vi "testVideo.vi"() -> ()   [LabVIEW 2009, in "run.lvlib"]
uses:
  run.lvlib
panel:
  out "Image":T1(plugin-control)
  in  "stop":bool
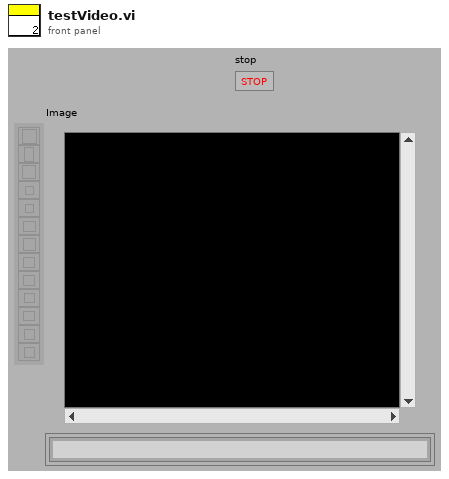
[diagram p1: front panel]
types:
  T1 = typedef "IMAQ Image.ctl" = refnum<image>
  T2 = typedef "Image Type" = u32
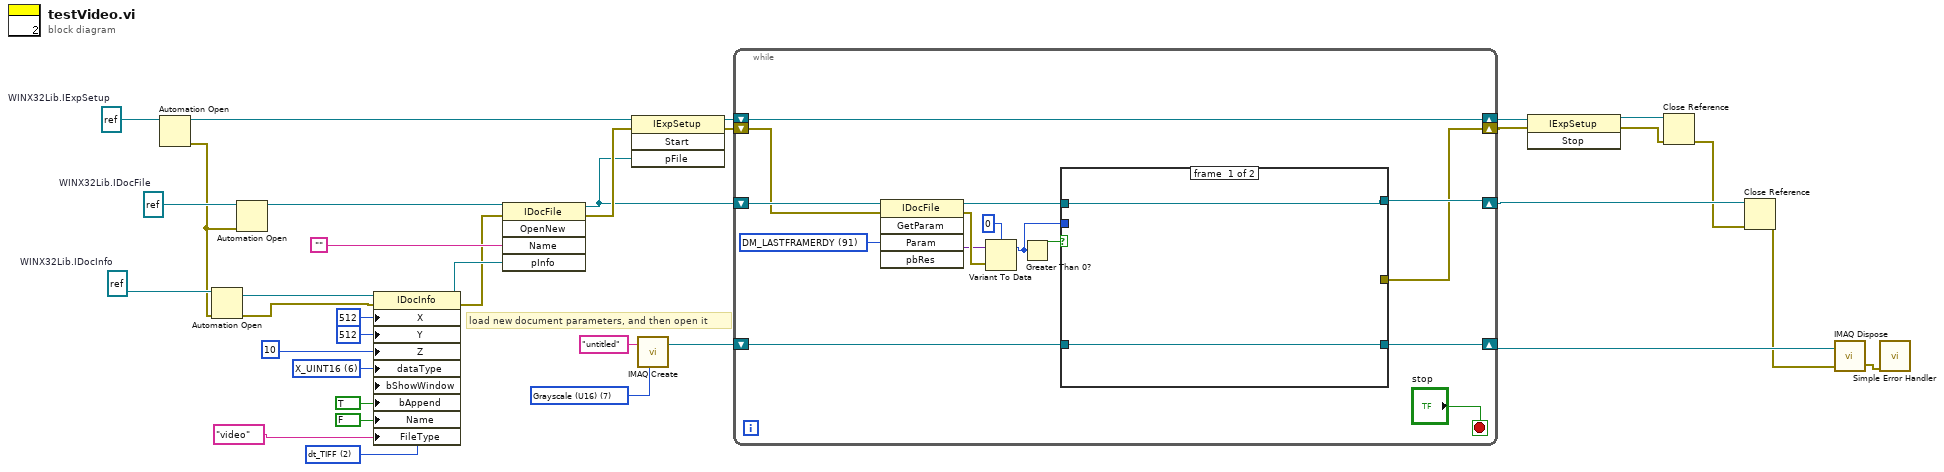
[diagram p0: block diagram]
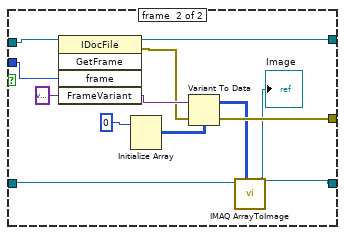
[diagram p2: hidden frame]
diagram:
  w10 = T2 7 items=["Grayscale (U8)", "Grayscale (I16)", "Grayscale (SGL)", "Complex (CSG)", "RGB (U32)", "HSL (U32)", "RGB (U64)", "Grayscale (U16)"] ("Image Type")
  w24 = refnum<k7> refnum  # WINX32Lib.IDocFile
  w28 = refnum<k7> refnum  # WINX32Lib.IDocInfo
  w31 = 6 items=["X_UNKNOWN"=0, "X_SHORT"=1, "X_LONG"=2, "X_FLOAT"=3, "X_DOUBLE"=4, "X_BYTE"=5, "X_UINT16"=6, "X_ULONG"=7, "X_LASTTYPE"=8, "X_ENUM"=9, "X_NODATATYPE"=10, "X_BOOL"=11, "X_CHAR_PTR"=13] ("dataType")
  w34 = 2 items=["dt_NONE", "dt_SPE", "dt_TIFF", "dt_TIF8", "dt_ASCII", "dt_NUMTYPES"] ("FileType")
  w35 = refnum<k7> refnum  # WINX32Lib.IExpSetup
  # "load new document parameters, and then open it"
  n1 = Automation Open(Automation Refnum=w35) -> (Automation Refnum=w17:refnum<k7>, error out=w23:errorcluster)  [unwired: 3 in]
  n2 = Automation Open(error in (no error)=w23, Automation Refnum=w28) -> (Automation Refnum=w27:refnum<k7>, error out=w26:errorcluster)  [unwired: 2 in]
  n3 = Automation Open(error in (no error)=w23, Automation Refnum=w24) -> (Automation Refnum=w21:refnum<k7>)  [unwired: 2 in, 1 out]
  n4 = property class="IDocInfo"(reference=w27, error in=w26, "X"=512, "Y"=512, "Z"=10, "dataType"=w31, "bShowWindow"=TRUE, "bAppend"=FALSE, "Name"="video", "FileType"=w34) -> (reference out=w20:refnum<k7>, error out=w19:errorcluster)
  n5 = invoke class="IDocFile" method="OpenNew"(reference=w21, error in=w19, "Name"="", "pInfo"=w20) -> (reference out=w13:refnum<k7>, error out=w14:errorcluster)  [unwired: 1 in, 3 out]
  n6 = invoke class="IExpSetup" method="Start"(reference=w17, error in=w14, "pFile"=w13) -> (reference out=w16:refnum<k7>, error out=w15:errorcluster)  [unwired: 1 in, 2 out]
  n7 = call "IMAQ Create"("Image Name"="untitled", "Image Type"=w10) -> ("New Image"=w11:T1)  [unwired: 3 in, 1 out]
  n8 = while {
    shift-right: [w39] -> w9
    shift-left: w16 -> [w39]
    shift-right: [w40] -> w8
    shift-left: w15 -> [w48]
    shift-right: [w41] -> w5
    shift-left: w13 -> [w50]
    shift-right: [w36] -> w3
    shift-left: w11 -> [w37]
    stop <- "stop" stop-if-true
    w49 = 91 items=["DM_XDIMDET"=1, "DM_YDIMDET"=2, "DM_TIMINGMODE"=3, "DM_EXPOSEC"=4, "DM_DETTYPE"=5, "DM_XDIM"=6, "DM_YDIM"=7, "DM_ASYNEN"=8, "DM_DATATYPE"=9, "DM_PIXELSIZE"=10, "DM_MINBLK"=11, "DM_NUMMINBLK"=12, "DM_ADCRATE"=13, "DM_ADCTYPE"=14, "DM_ADCRESOLUTION"=15, "DM_ADCBITADJUST"=16, "DM_GAIN"=17, "DM_GEOMETRIC"=18, "DM_CLEANS"=19, "DM_NUMSKPPERCLN"=20, "DM_FILEVERSION"=21, "DM_SWVERSION"=22, "DM_CONTROLLERTYPE"=23, "DM_NUMFRAMES"=24, "DM_MAXINTENSITY"=25, "DM_MININTENSITY"=26, "DM_SHUTTERTYPE"=27, "DM_SHUTTERCOMP"=28, "DM_READOUTMODE"=29, "DM_WINDOWSIZE"=30, "DM_CLKSPD"=31, "DM_KINTRIGMODE"=32, "DM_CLKSPD_us"=33, "DM_INTERFACETYPE"=34, "DM_NOT_IN_USE_0"=35, "DM_NOT_IN_USE_1"=36, "DM_NOT_IN_USE_2"=37, "DM_NOT_IN_USE_3"=38, "DM_NOT_IN_USE_4"=39, "DM_NOT_IN_USE_5"=40, "DM_COSMICAPPLIED"=41, "DM_COSMICTYPE"=42, "DM_COSMICTHRESHOLD"=43, "DM_BLEMISHAPPLIED"=44, "DM_FLATFIELDAPPLIED"=45, "DM_BACKGROUNDAPPLIED"=46, "DM_ACCUMS"=47, "DM_HWACCUMS"=48, "DM_NOT_IN_USE_6"=49, "DM_NOT_IN_USE_7"=50, "DM_NOT_IN_USE_8"=51, "DM_STORESYNC"=52, "DM_SWMADE"=53, "DM_FLATFIELDNAME"=54, "DM_BACKSUBNAME"=55, "DM_XLABEL"=56, "DM_YLABEL"=57, "DM_DLABEL"=58, "DM_FILEDATE"=59, "DM_BLEMISHFILE"=60, "DM_USERINFO"=61, "DM_USERCOMMENT1"=62, "DM_USERCOMMENT2"=63, "DM_USERCOMMENT3"=64, "DM_USERCOMMENT4"=65, "DM_USERCOMMENT5"=66, "DM_xCAL_OFFSET"=67, "DM_xCAL_FACTOR"=68, "DM_xCAL_CURR_UNIT"=69, "DM_xCAL_STRING"=70, "DM_xCAL_VALID"=71, "DM_xCAL_INPUT_UNIT"=72, "DM_xCAL_POLYNOM_UNIT"=73, "DM_xCAL_CALIB_COUNT"=74, "DM_xCAL_PXL_POS"=75, "DM_xCAL_PXL_VAL"=76, "DM_xCAL_POLYNOM_ORDER"=77, "DM_xCAL_COEFFS"=78, "DM_xCAL_LASERLINE"=79, "DM_xCAL_FILE_LABEL"=80, "DM_NUMROI"=81, "DM_ROI_STARTX"=82, "DM_ROI_ENDX"=83, "DM_ROI_GP_X"=84, "DM_ROI_STARTY"=85, "DM_ROI_ENDY"=86, "DM_ROI_GP_Y"=87, "DM_CONTROLLERNUM"=88, "DM_DEFAULTTYPE"=89, "DM_FRAMECOUNT"=90, "DM_LASTFRAMERDY"=91, "DM_FRAMEINPROS"=92, "DM_SCANCOUNT"=93, "DM_TEMPFLAG"=94, "DM_STOREFLAG"=95, "DM_FRAMESIZE"=96, "DM_ISDISPLAYED"=97, "DM_INUSE"=98, "DM_LASTVALUE"=99, "DM_STOREFLAGSAVE"=100, "DM_YTFLAG"=101, "DM_YT_AREAS_EQUS"=102, "DM_YT_POINTS_TAKEN"=103, "DM_FILENAME"=104, "DM_FILETITLE"=105, "DM_DOCTYPE"=106, "DM_NUMEXPREPEATS"=107, "DM_NUMEXPACCUMS"=108, "DM_UPDATEVIEWS"=109, "DM_PULSEFILENAME"=110, "DM_PULSEREPWIDTH"=111, "DM_PULSEREPDELAY"=112, "DM_CONTROLLERVERSION"=113, "DM_LOGICOUTPUT"=114, "DM_VIRTUALCHIPFLAG"=115, "DM_PULSERTYPE"=116, "DM_AMPHICAPLOWNOISE"=117, "DM_VCHIPXDIM"=118, "DM_VCHIPYDIM"=119, "DM_PIMAXUSED"=120, "DM_PIMAXMODE"=121, "DM_SHUTTERCONTROL"=122, "DM_ABSORBLIVE"=123, "DM_ABSORBMODE"=124, "DM_ABSORBSTRIPNUM"=125, "DM_THRESHOLDMINLIVE"=126, "DM_THRESHOLDMAXLIVE"=127, "DM_SPECAUTOSPECTROMODE"=128, "DM_SPECGLUEFLAG"=129, "DM_PULSERMODE"=130, "DM_PULSERONCHIPACCUMS"=131, "DM_PULSERREPEATEXP"=132, "DM_PULSESEQINCMODE"=133, "DM_ADCOFFSET"=134, "DM_ABSORBFILENAME"=135, "DM_NUMROISINEXPERIMENT"=136, "DM_SPECMIRRORLOCATION"=137, "DM_SPECSLITLOCATION"=138, "DM_SPECMIRRORPOS"=139, "DM_READOUTTIME"=140, "DM_DETTEMPERATURE"=141, "DM_DELAYTIME"=142, "DM_THRESHOLDMINVAL"=143, "DM_THRESHOLDMAXVAL"=144, "DM_SPECCENTERWLNM"=145, "DM_SPECGLUESTARTWLNM"=146, "DM_SPECGLUEENDWLNM"=147, "DM_SPECGLUEMINOVRLPNM"=148, "DM_SPECGLUEFINALRESNM"=149, "DM_PULSESEQSTARTWIDTH"=150, "DM_PULSESEQENDWIDTH"=151, "DM_PULSESEQSTARTDELAY"=152, "DM_PULSESEQENDDELAY"=153, "DM_SPECSLITPOS"=154, "DM_AUTOCLEANSACTIVE"=155, "DM_USECONTCLEANSINST"=156, "DM_CUSTOMCHIPFLAG"=157, "DM_XPREPIXELS"=158, "DM_XPOSTPIXELS"=159, "DM_YPREPIXELS"=160, "DM_YPOSTPIXELS"=161, "DM_CUSTOMTIMINGFLAG"=162, "DM_CANDOVIRTUALCHIPFLAG"=163, "DM_PIMAXGAIN"=164, "DM_PIMAX2NSBRDUSED"=165, "DM_TRIGGEREDMODEFLAG"=166, "DM_CONTINUOUSCLEANSFLAG"=167, "DM_EXTERNALTRIGGERFLAG"=168, "DM_EXPERIMENTTIMELOCAL"=169, "DM_EXPERIMENTTIMEUTC"=170, "DM_EXPOSUNITS"=171, "DM_SPECSLITPOSUNITS"=172, "DM_SPECGROOVES"=173, "DM_AVGAINUSED"=174, "DM_AVGAIN"=175, "DM_ANALOGGAIN"=176, "DM_SPECTYPE"=177, "DM_SPECMODEL"=178, "DM_PULSEBURSTUSED"=179, "DM_PULSEBURSTCOUNT"=180, "DM_PULSEBURSTPERIOD"=181, "DM_PULSEBRACKETUSED"=182, "DM_PULSEBRACKETTYPE"=183, "DM_PULSETIMECONSTFAST"=184, "DM_PULSEAMPLITUDEFAST"=185, "DM_PULSETIMECONSTSLOW"=186, "DM_PULSEAMPLITUDESLOW"=187] ("Param")
    n9 = invoke class="IDocFile" method="GetParam"(reference=w50, error in=w48, "Param"=w49) -> (reference out=w44:refnum<k7>, error out=w47:errorcluster, "GetParam"=w46:variant)  [unwired: 2 in, 2 out]
    n10 = Variant To Data(error in=w47, Variant=w46, type=0) -> (data=w42:i32)  [unwired: 1 out]
    n11 = Greater Than 0?(x=w42) -> (x > 0?=w43:bool)
    n12 = case shown="True" w43 {
      tunnel: w44 -> [w52 w64]
      tunnel: w42 -> [_ w63]
      tunnel: [w52 w57] -> w41
      tunnel: [_ w56] -> w40
      tunnel: w37 -> [w51 w55]
      tunnel: [w51 w53] -> w36
      frame #0 {
      }
      frame #1 {
        n13 = invoke class="IDocFile" method="GetFrame"(reference=w64, "frame"=w63, "FrameVariant"=variant) -> (reference out=w57:refnum<k7>, error out=w58:errorcluster, "FrameVariant"=w59:variant)  [unwired: 2 in, 2 out]
        n14 = Initialize Array(u16 0) -> (w60:u16[][])  [unwired: 2 in]
        n15 = Variant To Data(error in=w58, Variant=w59, type=w60) -> (error out=w56:errorcluster, data=w54:u16[][])
        n16 = call "IMAQ ArrayToImage"("Image Pixels (U16)"=w54, "Image"=w55) -> ("Image Out"=w53:T1)  [unwired: 8 in, 1 out]
        "Image" <- w53
      }
    }
  }
  n17 = invoke class="IExpSetup" method="Stop"(reference=w9, error in=w8) -> (reference out=w7:refnum<k7>, error out=w6:errorcluster)  [unwired: 1 in, 1 out]
  n18 = Close Reference(reference=w7, error in (no error)=w6) -> (error out=w4:errorcluster)
  n19 = Close Reference(reference=w5, error in (no error)=w4) -> (error out=w2:errorcluster)
  n20 = call "IMAQ Dispose"("Image"=w3, "error in (no error)"=w2) -> ("error out"=w1:errorcluster)  [unwired: 4 in]
  n21 = call <vilib>:"Simple Error Handler.vi"("error in (no error)"=w1) -> ()  [unwired: 4 in, 5 out]
